vi "observacao_queued.vi"() -> ()   [LabVIEW 2012, in "Shared_160.lvlib"] (continued)
                        n2703 = Greater?(x=w3327, y=w3326) -> (0:w3321:bool)
                        n2704 = case shown="True" w3321 {
                          frame False {
                          }
                          frame True {
                            n2705 = local write "LED ACTION"(TRUE ("LED ACTION")) -> ()
                          }
                        }
                        n2706 = Select(t="REPOUSO" ("y"), s=w3321, f="ESPERA3" ("y")) -> (s? t:f=w3324:string)
                      }
                      frame "REPOUSO" {
                      }
                    }
                    n2707 = local write "ESTADO ABRIR"(w3268) -> ()
                  }
                }
              }
              frame #2 {
                # "MÁQUINA DE ESTADOS PROTEÇÃO"
                n2708 = case shown="3" "M_PROT" {
                  selector: "M_PROT" -> [w3385 _ _ _ _ _]
                  tunnel: [w3385 w3386 w3405 5 5 ("estadoCUP") 0 ("estadoCUP")] -> w3383
                  frame 0, Default {
                    # "Sem movimento"
                    n2709 = call "TickTimeout.vi"() -> ("msTick"=→"Timeout PROT":u32)  [unwired: 2 in, 2 out]
                  }
                  frame 1 {
                    w3389 = u16 3 items=["Alarme", "Atencao", "Erro", "Ocupado", "Protecao", "Embreagem", "Tracking", "Var. Track", "Rápido", "Ligeiro", "Médio", "Lento", "Em movimento", ""] ("NomeStatus")
                    w3388 = u16 3 items=["Alarme", "Atencao", "Erro", "Ocupado", "Protecao", "Embreagem", "Tracking", "Var. Track", "Rápido", "Ligeiro", "Médio", "Lento", "Em movimento", ""] ("NomeStatus")
                    # "Testa Ocupado"
                    n2710 = call "Bit Status DEC.vi"("NomeStatus"=w3388) -> ("StatBit"=w3390:bool)
                    n2711 = call "Bit Status AH.vi"("NomeStatus"=w3389) -> ("StatBit"=w3391:bool)
                    n2712 = Or(x=w3391, y=w3390) -> (x .or. y?=w3387:bool)
                    n2713 = case shown="False" w3387 {
                      tunnel: [2 w3402] -> w3386
                      frame False {
                        w3398 = u16 2 items=["ZERO", "AH", "DEC", "TUBO", "CUP"] ("Controlador")
                        w3393 = u16 1 items=["ZERO", "AH", "DEC", "TUBO", "CUP"] ("Controlador")
                        # "Comando para os controladores\nsaírem da Proteção"
                        n2714 = call "Monta Comando.vi"("Comando"="LIBERAR", "Dispositivo"="EIXO" ("Comando"), "Controlador"=w3393) -> ()  [unwired: 4 in, 3 out]
                        n2715 = call "Monta Comando.vi"("Comando"="LIBERAR", "Dispositivo"="EIXO" ("Comando"), "Controlador"=w3398) -> ()  [unwired: 4 in, 3 out]
                      }
                      frame True {
                        # "Busy"
                        n2716 = local read "Timeout PROT"() -> (w3401:u32)
                        n2717 = call "TickTimeout.vi"("msInicial"=w3401, "msTimeout"=u32 20000) -> ("Timeout"=w3399:bool)  [unwired: 2 out]
                        n2718 = case shown="False" w3399 {
                          tunnel: [1 3] -> w3402
                          frame False {
                          }
                          frame True {
                          }
                        }
                      }
                    }
                  }
                  frame 2 {
                    # "Cálculos rápidos"
                    # "Vem do Setup"
                    # "Aguarda Sair da proteção"
                    n2719 = global read "Global_Telescopio.vi" "Zenital angle GRAUS"() -> (w3408:dbl)
                    n2720 = global read "Global_Telescopio.vi" "Z_LIBERA_GRAUS"() -> (w3407:dbl)
                    n2721 = Less?(x=w3408, y=w3407) -> (x < y?=w3406:bool)
                    n2722 = case shown="True" w3406 {
                      tunnel: [2 ("estadoCUP") 4 ("estadoCUP")] -> w3405
                      frame False {
                      }
                      frame True {
                        # "stop"
                      }
                    }
                  }
                  frame 3 {
                    w3411 = "TENTE NOVAMENTE" ("SYSTEM MESSAGES")
                    # "Trata Timeout"
                    n2723 = call "TickTimeout.vi"() -> ("msTick"=w3412:u32)  [unwired: 2 in, 2 out]
                    n2724 = call "Monta_Mensagem.vi"("Mensagem"=w3411) -> ()  [unwired: 2 in]
                    n2725 = call "Salva_systems_messages.vi"("Mensagem"=w3411) -> ()  [unwired: 5 in]
                    n2726 = local write "Timeout PROT"(w3412) -> ()
                  }
                  frame 4 {
                    w3415 = u16 1 items=["ZERO", "AH", "DEC", "TUBO", "CUP"] ("Controlador")
                    w3420 = u16 2 items=["ZERO", "AH", "DEC", "TUBO", "CUP"] ("Controlador")
                    # "Para os motores"
                    n2727 = call "Monta Comando.vi"("Comando"="PARAR", "Dispositivo"="PROG", "Controlador"=w3415) -> ()  [unwired: 4 in, 3 out]
                    n2728 = call "Monta Comando.vi"("Comando"="PARAR", "Dispositivo"="PROG", "Controlador"=w3420) -> ()  [unwired: 4 in, 3 out]
                  }
                  frame 5 {
                    # "SAÍDA"
                  }
                }
                n2729 = local write "M_PROT"(w3383) -> ()
              }
              frame #3 {
                w3439 = u16 3 items=["Alarme", "Atencao", "Erro", "Ocupado", "TBD", "LCB", "Trapeira", "Paravento", "DomoRap", "DomoCW", "DomoCCW", "TBD", "Em movimento", "TBD"] ("NomeStatus")
                w3447 = u16 3 items=["Alarme", "Atencao", "Erro", "Ocupado", "Protecao", "Embreagem", "Tracking", "Var. Track", "Rápido", "Ligeiro", "Médio", "Lento", "Em movimento", ""] ("NomeStatus")
                w3448 = u16 3 items=["Alarme", "Atencao", "Erro", "Ocupado", "Protecao", "Embreagem", "Tracking", "Var. Track", "Rápido", "Ligeiro", "Médio", "Lento", "Em movimento", ""] ("NomeStatus")
                n2730 = global read "Global_Telescopio.vi" "LimiarRapMed"() -> (w3449:dbl)
                n2731 = global read "Global_Telescopio.vi" "PosAH"() -> (w3451:dbl)
                n2732 = global read "Global_Telescopio.vi" "ErroMaxEixo"() -> (w3446:dbl)
                n2733 = global read "Global_Telescopio.vi" "PosDEC"() -> (w3450:dbl)
                n2734 = call "Bit Status DEC.vi"("NomeStatus"=w3447) -> ("StatBit"=w3445:bool)
                n2735 = call "Bit Status AH.vi"("NomeStatus"=w3448) -> ("StatBit"=w3444:bool)
                n2736 = case shown="4" "M_DEC" {
                  selector: "M_DEC" -> [w3548 _ _ _ _ _ _ _ _]
                  tunnel: [w3548 w3554 w3581 w3606 w3629 w3653 0 w3670 w3675] -> w3428
                  tunnel: "DestDEC" -> [_ w3553 w3578 w3600 w3626 _ _ _ _]
                  tunnel: w3450 -> [_ w3556 _ w3603 _ _ _ _ _]
                  tunnel: w3446 -> [_ _ _ w3604 _ _ _ _ _]
                  tunnel: w3449 -> [_ w3555 _ _ _ _ _ _ _]
                  tunnel: w3445 -> [_ w3552 _ w3599 _ _ _ _ _]
                  frame 0, Default {
                    w3546 = 0 ("CR DEC")
                    # "Sem apontamento"
                    n2737 = call "TickTimeout.vi"() -> ("msTick"=→"TimeoutDEC 2":u32)  [unwired: 2 in, 2 out]
                    "CR DEC UTILS" <- w3546
                    "CONT DEC UTILS" <- w3546
                  }
                  frame 1 {
                    # "Envia\nComando"
                    n2738 = Subtract(x=w3553, y=w3556) -> (x-y=w3551:dbl)
                    n2739 = Absolute Value(x=w3551) -> (abs(x)=w3557:dbl)
                    n2740 = Less?(x=w3557, y=w3555) -> (x < y?=w3550:bool)
                    n2741 = case shown="False" w3550 {
                      tunnel: [w3561 3] -> w3554
                      tunnel: w3553 -> [w3560 _]
                      tunnel: w3551 -> [w3559 _]
                      tunnel: w3552 -> [w3558 _]
                      frame False {
                        # "destino"
                        # "Fora do"
                        n2742 = case shown="False" w3558 {
                          tunnel: [20 w3570] -> w3561
                          tunnel: w3560 -> [w3564 _]
                          tunnel: w3559 -> [_ _]
                          frame False {
                            w3568 = u16 2 items=["ZERO", "AH", "DEC", "TUBO", "CUP"] ("Controlador")
                            # "CLP Pronto"
                            n2743 = local write "DEC on Target"(FALSE ("DEC on Target")) -> ()
                            n2744 = call "rad_hms.vi"("TRUE=HORA\nFALSE=GRAU"=FALSE, "Radiano"=w3564) -> ("Hora/Graus Texto Decimal"=w3565:string)  [unwired: 3 in]
                            n2745 = call "Monta Comando.vi"("Set Point"=w3565, "Comando"="MOVER_RAP", "Dispositivo"="EIXO" ("Comando"), "Controlador"=w3568) -> ()  [unwired: 3 in, 3 out]
                          }
                          frame True {
                            # "CLP Ocupado"
                            n2746 = local read "TimeoutDEC 2"() -> (w3572:u32)
                            n2747 = call "TickTimeout.vi"("msInicial"=w3572, "msTimeout"=u32 4000) -> ("Timeout"=w3571:bool)  [unwired: 2 out]
                            n2748 = case shown="False" w3571 {
                              tunnel: [1 5] -> w3570
                              frame False {
                              }
                              frame True {
                                # "Tratar\nTimeout"
                              }
                            }
                          }
                        }
                      }
                      frame True {
                        # "Dist. pequena p/ mov. rápido"
                        # "Ligar mov. lento"
                        n2749 = call "TickTimeout.vi"() -> ("msTick"=w3576:u32)  [unwired: 2 in, 2 out]
                        n2750 = local write "TimeoutDEC 2"(w3576) -> ()
                      }
                    }
                    n2751 = local write "dec="(FALSE ("dec=")) -> ()
                  }
                  frame 2 {
                    w3584 = u16 12 items=["Alarme", "Atencao", "Erro", "Ocupado", "Protecao", "Embreagem", "Tracking", "Var. Track", "Rápido", "Ligeiro", "Médio", "Lento", "Em movimento", ""] ("NomeStatus")
                    # "Aguarda fim mov. Rap."
                    n2752 = call "Bit Status DEC.vi"("NomeStatus"=w3584) -> ("StatBit"=w3585:bool)
                    n2753 = case shown="True" w3585 {
                      tunnel: [1 w3594] -> w3582
                      tunnel: w3578 -> [_ w3593]
                      frame False {
                        # "Motor parado.\nTestar se chegou\nao destino"
                        n2754 = call "TickTimeout.vi"() -> ("msTick"=w3590:u32)  [unwired: 2 in, 2 out]
                        n2755 = local write "TimeoutDEC 2"(w3590) -> ()
                      }
                      frame True {
                        # "Ainda movendo...\nAGUARDAR"
                        n2756 = call "PROTECAO_DEC_UTILS.vi"("Destino DEC"=w3593) -> ("CONT DEC"=w3592:i32)  [unwired: 10 in]
                        n2757 = local read "Erro PROTEC"() -> (w3595:i32)
                        n2758 = Greater Or Equal?(x=w3592, y=w3595) -> (x >= y?=w3598:bool)
                        n2759 = local write "CONT DEC UTILS"(w3592) -> ()
                        n2760 = Select(t=6, s=w3598, f=2) -> (s? t:f=w3594:i32)
                      }
                    }
                    n2761 = global read "Global_Telescopio.vi" "Habilita supervisao"() -> (w3580:bool)
                    n2762 = case shown="True" w3580 {
                      tunnel: [FALSE w3589] -> w3579
                      frame False {
                      }
                      frame True {
                        n2763 = local read "CR DEC UTILS"() -> (w3587:i32)
                        n2764 = local read "Erro Lim"() -> (w3588:i32)
                        n2765 = Greater Or Equal?(x=w3587, y=w3588) -> (x >= y?=w3589:bool)
                      }
                    }
                    n2766 = Select(t=6, s=w3579, f=w3582) -> (s? t:f=w3581:i32)
                  }
                  frame 3 {
                    # "Mov.Lento"
                    n2767 = Subtract(x=w3600, y=w3603) -> (x-y=w3601:dbl)
                    n2768 = Absolute Value(x=w3601) -> (abs(x)=w3605:dbl)
                    n2769 = Less Or Equal?(x=w3605, y=w3604) -> (x <= y?=w3602:bool)
                    n2770 = case shown="False" w3602 {
                      tunnel: [w3608 0] -> w3606
                      tunnel: w3601 -> [w3607 _]
                      tunnel: w3599 -> [w3609 _]
                      frame False {
                        n2771 = case shown="False" w3609 {
                          tunnel: [40 w3618] -> w3608
                          tunnel: w3607 -> [w3612 _]
                          frame False {
                            w3617 = u16 2 items=["ZERO", "AH", "DEC", "TUBO", "CUP"] ("Controlador")
                            # "Mov. lento"
                            n2772 = call "TickTimeout.vi"() -> ("msTick"=w3610:u32)  [unwired: 2 in, 2 out]
                            n2773 = local write "TimeoutDEC 2"(w3610) -> ()
                            n2774 = call "rad_hms.vi"("TRUE=HORA\nFALSE=GRAU"=FALSE ("TRUE=HORA\nFALSE=GRAU"), "Radiano"=w3612) -> ("Hora/Graus Texto Decimal"=w3614:string)  [unwired: 3 in]
                            n2775 = call "Monta Comando.vi"("Set Point"=w3614, "Comando"="MOVER_REL", "Dispositivo"="EIXO" ("Comando"), "Controlador"=w3617) -> ()  [unwired: 3 in, 3 out]
                          }
                          frame True {
                            # "CLP Ocupado"
                            n2776 = local read "TimeoutDEC 2"() -> (w3620:u32)
                            n2777 = call "TickTimeout.vi"("msInicial"=w3620, "msTimeout"=u32 2000) -> ("Timeout"=w3619:bool)  [unwired: 2 out]
                            n2778 = case shown="False" w3619 {
                              tunnel: [3 5] -> w3618
                              frame False {
                              }
                              frame True {
                              }
                            }
                          }
                        }
                      }
                      frame True {
                        # "DEC no destino"
                        n2779 = local write "DEC on Target"(TRUE ("DEC on Target")) -> ()
                      }
                    }
                  }
                  frame 4 {
                    w3632 = u16 12 items=["Alarme", "Atencao", "Erro", "Ocupado", "Protecao", "Embreagem", "Tracking", "Var. Track", "Rápido", "Ligeiro", "Médio", "Lento", "Em movimento", ""] ("NomeStatus")
                    # "Aguarda fim mov. lento"
                    n2780 = call "Bit Status DEC.vi"("NomeStatus"=w3632) -> ("StatBit"=w3633:bool)
                    n2781 = case shown="True" w3633 {
                      tunnel: [3 w3643] -> w3628
                      tunnel: w3626 -> [_ w3641]
                      frame False {
                        # "Motor parado.\nTestar se chegou\nao destino"
                        n2782 = call "TickTimeout.vi"() -> ("msTick"=w3638:u32)  [unwired: 2 in, 2 out]
                        n2783 = local write "TimeoutDEC 2"(w3638) -> ()
                      }
                      frame True {
                        n2784 = call "PROTECAO_DEC_UTILS.vi"("Destino DEC"=w3641) -> ("CONT DEC"=w3640:i32)  [unwired: 10 in]
                        n2785 = local read "Erro PROTEC"() -> (w3646:i32)
                        n2786 = local write "CONT DEC UTILS"(w3640) -> ()
                        n2787 = Greater Or Equal?(x=w3640, y=w3646) -> (x >= y?=w3648:bool)
                        n2788 = local read "TimeoutDEC 2"() -> (w3642:u32)
                        n2789 = call "TickTimeout.vi"("msInicial"=w3642, "msTimeout"=u32 4000) -> ("Timeout"=w3645:bool)  [unwired: 2 out]
                        n2790 = case shown="False" w3645 {
                          tunnel: [4 5] -> w3649
                          frame False {
                          }
                          frame True {
                          }
                        }
                        n2791 = Select(t=6, s=w3648, f=w3649) -> (s? t:f=w3643:i32)
                      }
                    }
                    n2792 = global read "Global_Telescopio.vi" "Habilita supervisao"() -> (w3631:bool)
                    n2793 = case shown="True" w3631 {
                      tunnel: [FALSE w3637] -> w3627
                      frame False {
                      }
                      frame True {
                        n2794 = local read "CR DEC UTILS"() -> (w3635:i32)
                        n2795 = local read "Erro Lim"() -> (w3636:i32)
                        n2796 = Greater Or Equal?(x=w3635, y=w3636) -> (x >= y?=w3637:bool)
                      }
                    }
                    n2797 = Select(t=6, s=w3627, f=w3628) -> (s? t:f=w3629:i32)
                  }
                  frame 5 {
                    w3659 = u16 2 items=["ZERO", "AH", "DEC", "TUBO", "CUP"] ("Controlador")
                    # "Reiniciar apontamento"
                    # "Trata Timeout"
                    n2798 = call "TickTimeout.vi"() -> ("msTick"=w3652:u32)  [unwired: 2 in, 2 out]
                    n2799 = local write "TimeoutDEC 2"(w3652) -> ()
                    n2800 = call "Monta Comando.vi"("Comando"="PARAR", "Dispositivo"="PROG" ("Comando"), "Controlador"=w3659) -> ("Erro Comunicação"=w3654:bool)  [unwired: 4 in, 2 out]
                    n2801 = Select(t=6, s=w3654, f=1) -> (s? t:f=w3653:i32)
                  }
                  frame 6 {
                    n2802 = stacked-sequence {
                      frame #0 {
                        w3664 = u16 2 items=["ZERO", "AH", "DEC", "TUBO", "CUP"] ("Controlador")
                        # "Trata Timeout"
                        n2803 = local write "dec="(TRUE ("dec=")) -> ()
                        n2804 = call "Monta Comando.vi"("Comando"="PARAR", "Dispositivo"="PROG" ("Comando"), "Controlador"=w3664) -> ()  [unwired: 4 in, 3 out]
                      }
                      frame #1 {
                        w3666 = "Erro de Controlador DEC , REAPONTAR !" ("Mensagem")
                        n2805 = local write "Flag de erro p/ apagar lampada"(TRUE ("Flag de erro p/ apagar lampada")) -> ()
                        n2806 = call "Monta_Mensagem.vi"("Mensagem"=w3666) -> ()  [unwired: 2 in]
                        n2807 = call "Salva_systems_messages.vi"("Mensagem"=w3666) -> ()  [unwired: 5 in]
                      }
                      frame #2 {
                        w3668 = u16 2 items=["ZERO", "AH", "DEC", "TUBO", "CUP"] ("Controlador")
                        # "Em movimento não aceita reset"
                        # "Segundo PARAR por garantia"
                        n2808 = call "Monta Comando.vi"("Comando"="PARAR", "Dispositivo"="PROG", "Controlador"=w3668) -> ()  [unwired: 4 in, 3 out]
                      }
                    }
                  }
                  frame 20 {
                    # "Espera entrar\nem movimento"
                    n2809 = local read "Flag ativo DEC"() -> (w3671:bool)
                    n2810 = case shown="True" w3671 {
                      tunnel: [20 ("t") 2 ("t")] -> w3670
                      frame False {
                      }
                      frame True {
                        # "limpa flag"
                        n2811 = local write "Flag ativo DEC"(FALSE ("Flag ativo AH")) -> ()
                      }
                    }
                  }
                  frame 40 {
                    # "Espera entrar\nem movimento"
                    n2812 = local read "Flag ativo DEC"() -> (w3676:bool)
                    n2813 = case shown="True" w3676 {
                      tunnel: [40 ("t") 4 ("t")] -> w3675
                      frame False {
                      }
                      frame True {
                        # "limpa flag"
                        n2814 = local write "Flag ativo DEC"(FALSE ("Flag ativo AH")) -> ()
                      }
                    }
                  }
                }
                n2815 = case shown="1" "M_AH" {
                  selector: "M_AH" -> [w3682 _ _ _ _ _ _ _ _ _ _]
                  tunnel: [w3682 w3683 w3703 w3734 5 w3757 w3786 w3808 0 w3826 w3831] -> w3430
                  tunnel: "DestAH" -> [_ _ w3700 w3730 _ w3753 w3782 _ _ _ _]
                  tunnel: w3451 -> [_ _ w3706 _ _ w3759 _ _ _ _ _]
                  tunnel: w3446 -> [_ _ _ _ _ w3758 _ _ _ _ _]
                  tunnel: w3449 -> [_ _ w3707 _ _ _ _ _ _ _ _]
                  tunnel: w3444 -> [_ w3684 w3701 _ _ w3755 _ _ _ _ _]
                  frame 0, Default {
                    w3680 = 0 ("CR AH")
                    # "Sem apontamento"
                    n2816 = call "TickTimeout.vi"() -> ("msTick"=→"TimeoutAH 2":u32)  [unwired: 2 in, 2 out]
                    "CR AH UTILS" <- w3680
                    "CONT AH UTILS" <- w3680
                  }
                  frame 1 {
                    n2817 = case shown="False" w3684 {
                      tunnel: [2 w3694] -> w3683
                      frame False {
                        n2818 = stacked-sequence {
                          frame #0 {
                            w3689 = u16 1 items=["ZERO", "AH", "DEC", "TUBO", "CUP"] ("Controlador")
                            # "Desliga Acomp Sideral"
                            n2819 = call "Monta Comando.vi"("Comando"="DESLIGAR", "Dispositivo"="SIDERAL" ("Comando"), "Controlador"=w3689) -> ()  [unwired: 4 in, 3 out]
                          }
                          frame #1 {
                            w3692 = u16 1 items=["ZERO", "AH", "DEC", "TUBO", "CUP"] ("Controlador")
                            # "Parar Eixo AH"
                            n2820 = call "Monta Comando.vi"("Comando"="PARAR", "Dispositivo"="PROG" ("Comando"), "Controlador"=w3692) -> ()  [unwired: 4 in, 3 out]
                          }
                        }
                        n2821 = call "TickTimeout.vi"() -> ("msTick"=w3685:u32)  [unwired: 2 in, 2 out]
                        n2822 = local write "TimeoutAH 2"(w3685) -> ()
                      }
                      frame True {
                        n2823 = local read "TimeoutAH 2"() -> (w3693:u32)
                        n2824 = call "TickTimeout.vi"("msInicial"=w3693, "msTimeout"=u32 5000) -> ("Timeout"=w3696:bool)  [unwired: 2 out]
                        n2825 = case shown="False" w3696 {
                          tunnel: [1 7] -> w3694
                          frame False {
                          }
                          frame True {
                          }
                        }
                      }
                    }
                  }
                  frame 2 {
                    # "Mov.Rapido"
                    n2826 = Subtract(x=w3700, y=w3706) -> (x-y=w3704:dbl)
                    n2827 = Absolute Value(x=w3704) -> (abs(x)=w3705:dbl)
                    n2828 = Less?(x=w3705, y=w3707) -> (x < y?=w3702:bool)
                    n2829 = case shown="False" w3702 {
                      tunnel: w3700 -> [w3708 _]
                      tunnel: w3704 -> [_ _]
                      tunnel: [w3709 4] -> w3703
                      tunnel: w3701 -> [w3710 _]
                      frame False {
                        n2830 = case shown="False" w3710 {
                          tunnel: w3708 -> [w3716 _]
                          tunnel: [w3711 w3722] -> w3709
                          frame False {
                            w3718 = u16 1 items=["ZERO", "AH", "DEC", "TUBO", "CUP"] ("Controlador")
                            # "Aguardar\nfim mov."
                            # "Mov. rápido"
                            n2831 = local write "RA on Target"(FALSE ("RA on Target")) -> ()
                            n2832 = call "rad_hms.vi"("TRUE=HORA\nFALSE=GRAU"=TRUE ("TRUE=HORA\nFALSE=GRAU"), "Radiano"=w3716) -> ("Hora/Graus Texto Decimal"=w3721:string)  [unwired: 3 in]
                            n2833 = call "Monta Comando.vi"("Set Point"=w3721, "Comando"="MOVER_RAP", "Dispositivo"="EIXO" ("Comando"), "Controlador"=w3718) -> ("Erro Comunicação"=w3712:bool)  [unwired: 3 in, 2 out]
                            n2834 = Select(t=8, s=w3712, f=30) -> (s? t:f=w3711:i32)
                          }
                          frame True {
                            # "CLP Ocupado"
                            n2835 = local read "TimeoutAH 2"() -> (w3724:u32)
                            n2836 = call "TickTimeout.vi"("msInicial"=w3724, "msTimeout"=u32 4000) -> ("Timeout"=w3723:bool)  [unwired: 2 out]
                            n2837 = case shown="True" w3723 {
                              tunnel: [2 7] -> w3722
                              frame False {
                              }
                              frame True {
                                # "Tratar\nTimeout"
                              }
                            }
                          }
                        }
                      }
                      frame True {
                        # "Dist. pequena p/ mov. rápido"
                        n2838 = call "TickTimeout.vi"() -> ("msTick"=w3728:u32)  [unwired: 2 in, 2 out]
                        n2839 = local write "TimeoutAH 2"(w3728) -> ()
                      }
                    }
                    n2840 = local write "ah="(FALSE ("ah=")) -> ()
                  }
                  frame 3 {
                    w3737 = u16 12 items=["Alarme", "Atencao", "Erro", "Ocupado", "Protecao", "Embreagem", "Tracking", "Var. Track", "Rápido", "Ligeiro", "Médio", "Lento", "Em movimento", ""] ("NomeStatus")
                    # "Aguarda fim mov. Rap."
                    n2841 = call "Bit Status AH.vi"("NomeStatus"=w3737) -> ("StatBit"=w3736:bool)
                    n2842 = case shown="True" w3736 {
                      tunnel: [2 w3746] -> w3733
                      tunnel: w3730 -> [_ w3745]
                      frame False {
                        # "Motor parado.\nTestar se precisa\nde novo cmd. \nde mov. rápido"
                        n2843 = call "TickTimeout.vi"() -> ("msTick"=w3742:u32)  [unwired: 2 in, 2 out]
                        n2844 = local write "TimeoutAH 2"(w3742) -> ()
                      }
                      frame True {
                        # "Aqui também \ncaberia um \nTimeout?"
                        # "Ainda movendo...\nAGUARDAR"
                        n2845 = call "PROTECAO_AH_UTILS.vi"("DestinoAH"=w3745) -> ("CONT AH"=w3744:i32)  [unwired: 10 in]
                        n2846 = local read "Erro PROTEC"() -> (w3748:i32)
                        n2847 = local write "CONT AH UTILS"(w3744) -> ()
                        n2848 = Greater Or Equal?(x=w3744, y=w3748) -> (x >= y?=w3749:bool)
                        n2849 = Select(t=8, s=w3749, f=3) -> (s? t:f=w3746:i32)
                      }
                    }
                    n2850 = global read "Global_Telescopio.vi" "Habilita supervisao"() -> (w3732:bool)
                    n2851 = case shown="True" w3732 {
                      tunnel: [FALSE w3741] -> w3731
                      frame False {
                      }
                      frame True {
                        n2852 = local read "Erro Lim"() -> (w3740:i32)
                        n2853 = local read "CR AH UTILS"() -> (w3739:i32)
                        n2854 = Greater Or Equal?(x=w3739, y=w3740) -> (x >= y?=w3741:bool)
                      }
                    }
                    n2855 = Select(t=8, s=w3731, f=w3733) -> (s? t:f=w3734:i32)
                  }
                  frame 4 {
                    # "Não faz nada"
                    n2856 = call "TickTimeout.vi"() -> ("msTick"=w3752:u32)  [unwired: 2 in, 2 out]
                    n2857 = local write "TimeoutAH 2"(w3752) -> ()
                  }
                  frame 5 {
                    # "Mov.Lento"
                    n2858 = Subtract(x=w3753, y=w3759) -> (x-y=w3754:dbl)
                    n2859 = Absolute Value(x=w3754) -> (abs(x)=w3760:dbl)
                    n2860 = Less Or Equal?(x=w3760, y=w3758) -> (x <= y?=w3756:bool)
                    n2861 = case shown="True" w3756 {
                      tunnel: w3754 -> [w3762 _]
                      tunnel: [w3761 0] -> w3757
                      tunnel: w3755 -> [w3763 _]
                      frame False {
                        n2862 = case shown="False" w3763 {
                          tunnel: w3762 -> [w3768 _]
                          tunnel: [w3767 w3774] -> w3761
                          frame False {
                            w3770 = u16 1 items=["ZERO", "AH", "DEC", "TUBO", "CUP"] ("Controlador")
                            # "Envia Cmd. Mov. Lento"
                            n2863 = call "rad_hms.vi"("TRUE=HORA\nFALSE=GRAU"=TRUE ("TRUE=HORA\nFALSE=GRAU"), "Radiano"=w3768) -> ("Hora/Graus Texto Decimal"=w3773:string)  [unwired: 3 in]
                            n2864 = call "Monta Comando.vi"("Set Point"=w3773, "Comando"="MOVER_REL", "Dispositivo"="EIXO" ("Comando"), "Controlador"=w3770) -> ("Erro Comunicação"=w3765:bool)  [unwired: 3 in, 2 out]
                            n2865 = Select(t=8, s=w3765, f=60) -> (s? t:f=w3767:i32)
                          }
                          frame True {
                            # "CLP Ocupado"
                            n2866 = local read "TimeoutAH 2"() -> (w3776:u32)
                            n2867 = call "TickTimeout.vi"("msInicial"=w3776, "msTimeout"=u32 4000) -> ("Timeout"=w3775:bool)  [unwired: 2 out]
                            n2868 = case shown="False" w3775 {
                              tunnel: [5 7] -> w3774
                              frame False {
                              }
                              frame True {
                              }
                            }
                          }
                        }
                      }
                      frame True {
                        # "AH on Target"
                        n2869 = local write "RA on Target"(TRUE ("RA on Target")) -> ()
                      }
                    }
                  }
                  frame 6 {
                    w3789 = u16 12 items=["Alarme", "Atencao", "Erro", "Ocupado", "Protecao", "Embreagem", "Tracking", "Var. Track", "Rápido", "Ligeiro", "Médio", "Lento", "Em movimento", ""] ("NomeStatus")
                    # "Aguarda fim mov. Lento"
                    n2870 = call "Bit Status AH.vi"("NomeStatus"=w3789) -> ("StatBit"=w3788:bool)
                    n2871 = case shown="True" w3788 {
                      tunnel: [5 w3803] -> w3785
                      tunnel: w3782 -> [_ w3797]
                      frame False {
                        # "Motor parado.\nTestar se chegou\nao destino"
                        n2872 = call "TickTimeout.vi"() -> ("msTick"=w3794:u32)  [unwired: 2 in, 2 out]
                        n2873 = local write "TimeoutAH 2"(w3794) -> ()
                      }
                      frame True {
                        n2874 = local read "Erro PROTEC"() -> (w3805:i32)
                        n2875 = call "PROTECAO_AH_UTILS.vi"("DestinoAH"=w3797) -> ("CONT AH"=w3796:i32)  [unwired: 10 in]
                        n2876 = local write "CONT AH UTILS"(w3796) -> ()
                        n2877 = local read "TimeoutAH 2"() -> (w3798:u32)
                        n2878 = Greater Or Equal?(x=w3796, y=w3805) -> (x >= y?=w3799:bool)
                        n2879 = call "TickTimeout.vi"("msInicial"=w3798, "msTimeout"=u32 4000) -> ("Timeout"=w3802:bool)  [unwired: 2 out]
                        n2880 = case shown="False" w3802 {
                          tunnel: [6 7] -> w3800
                          frame False {
                          }
                          frame True {
                            # "Tratar\nTimeout"
                          }
                        }
                        n2881 = Select(t=8, s=w3799, f=w3800) -> (s? t:f=w3803:i32)
                      }
                    }
                    n2882 = global read "Global_Telescopio.vi" "Habilita supervisao"() -> (w3784:bool)
                    n2883 = case shown="True" w3784 {
                      tunnel: [FALSE w3793] -> w3783
                      frame False {
                      }
                      frame True {
                        n2884 = local read "CR AH UTILS"() -> (w3791:i32)
                        n2885 = local read "Erro Lim"() -> (w3792:i32)
                        n2886 = Greater Or Equal?(x=w3791, y=w3792) -> (x >= y?=w3793:bool)
                      }
                    }
                    n2887 = Select(t=8, s=w3783, f=w3785) -> (s? t:f=w3786:i32)
                  }
                  frame 7 {
                    w3813 = u16 1 items=["ZERO", "AH", "DEC", "TUBO", "CUP"] ("Controlador")
                    # "Reiniciar apontamento"
                    # "Trata Timeout"
                    n2888 = call "TickTimeout.vi"() -> ("msTick"=w3812:u32)  [unwired: 2 in, 2 out]
                    n2889 = local write "TimeoutAH 2"(w3812) -> ()
                    n2890 = call "Monta Comando.vi"("Comando"="PARAR", "Dispositivo"="PROG" ("Comando"), "Controlador"=w3813) -> ("Erro Comunicação"=w3809:bool)  [unwired: 4 in, 2 out]
                    n2891 = Select(t=8, s=w3809, f=2) -> (s? t:f=w3808:i32)
                  }
                  frame 8 {
                    n2892 = stacked-sequence {
                      frame #0 {
                        w3818 = u16 1 items=["ZERO", "AH", "DEC", "TUBO", "CUP"] ("Controlador")
                        # "Reiniciar apontamento"
                        # "Trata Timeout"
                        n2893 = local write "ah="(TRUE ("ah=")) -> ()
                        n2894 = call "Monta Comando.vi"("Comando"="PARAR", "Dispositivo"="PROG" ("Comando"), "Controlador"=w3818) -> ()  [unwired: 4 in, 3 out]
                      }
                      frame #1 {
                        w3822 = "Erro de Controlador RA , REAPONTAR !" ("Mensagem")
                        n2895 = local write "Flag de erro p/ apagar lampada"(TRUE ("Flag de erro p/ apagar lampada")) -> ()
                        n2896 = call "Monta_Mensagem.vi"("Mensagem"=w3822) -> ()  [unwired: 2 in]
                        n2897 = call "Salva_systems_messages.vi"("Mensagem"=w3822) -> ()  [unwired: 5 in]
                      }
                      frame #2 {
                        w3825 = u16 1 items=["ZERO", "AH", "DEC", "TUBO", "CUP"] ("Controlador")
                        # "Em movimento não aceita reset"
                        # "Segundo PARAR por garantia"
                        n2898 = call "Monta Comando.vi"("Comando"="PARAR", "Dispositivo"="PROG", "Controlador"=w3825) -> ()  [unwired: 4 in, 3 out]
                      }
                    }
                  }
                  frame 30 {
                    # "Espera entrar\nem movimento"
                    n2899 = local read "Flag ativo AH"() -> (w3827:bool)
                    n2900 = case shown="True" w3827 {
                      tunnel: [30 ("t") 3 ("t")] -> w3826
                      frame False {
                      }
                      frame True {
                        # "limpa flag"
                        n2901 = local write "Flag ativo AH"(FALSE ("Flag ativo AH")) -> ()
                      }
                    }
                  }
                  frame 60 {
                    # "Espera entrar\nem movimento"
                    n2902 = local read "Flag ativo AH"() -> (w3832:bool)
                    n2903 = case shown="True" w3832 {
                      tunnel: [60 ("t") 6 ("t")] -> w3831
                      frame False {
                      }
                      frame True {
                        # "limpa flag"
                        n2904 = local write "Flag ativo AH"(FALSE ("Flag ativo AH")) -> ()
                      }
                    }
                  }
                }
                n2905 = call "PROTECAO.vi"("Estado In"=w3428) -> ("Estado Out"=w3427:i32)  [unwired: 2 in]
                n2906 = call "PROTECAO.vi"("Estado In"=w3430) -> ("Estado Out"=w3429:i32)  [unwired: 2 in]
                n2907 = local write "M_DEC"(w3427) -> ()
                n2908 = property on="Setup, Pointing & Guiding" class="TabCtl (strict)"() -> ("Page Selector Visible"=w3434:bool)  [unwired: 2 in, 2 out]
                n2909 = local write "M_AH"(w3429) -> ()
                n2910 = global read "Global_Telescopio.vi" "PosCUP"() -> (w3442:i16)
                n2911 = global read "Global_Telescopio.vi" "ErroMaxCup"() -> (w3441:i16)
                n2912 = local read "M_PROT"() -> (w3424:i32)
                n2913 = call "Bit Status CUP.vi"("NomeStatus"=w3439) -> ("StatBit"=w3443:bool)
                n2914 = Not(x=w3434) -> (.not. x?=w3432:bool)
                n2915 = case shown="5" "M_CUP" {
                  selector: "M_CUP" -> [w3456 _ _ _ _ _ _ _ _]
                  tunnel: [w3456 w3457 w3488 1 w3500 w3517 w3522 w3539 0 ("estadoCUP")] -> w3426
                  tunnel: w3443 -> [_ w3459 _ _ w3499 _ w3523 _ _]
                  tunnel: w3442 -> [_ w3463 _ _ _ _ _ _ _]
                  tunnel: "DestCUP" -> [_ w3458 _ _ _ _ _ _ _]
                  tunnel: w3441 -> [_ w3461 _ _ _ _ _ _ _]
                  frame 0, Default {
                    # "Sem movimento"
                    n2916 = call "TickTimeout.vi"() -> ("msTick"=→"TimeoutCUP 2":u32)  [unwired: 2 in, 2 out]
                  }
                  frame 1 {
                    # "Envia\nComando"
                    n2917 = Subtract(x=w3458, y=w3463) -> (x-y=w3462:i16)
                    n2918 = Absolute Value(x=w3462) -> (abs(x)=w3464:i16)
                    n2919 = Less Or Equal?(x=w3464, y=w3461) -> (x <= y?=w3460:bool)
                    n2920 = case shown="True" w3460 {
                      tunnel: w3459 -> [w3467 _]
                      tunnel: w3458 -> [w3466 _]
                      tunnel: [w3465 w3482] -> w3457
                      frame False {
                        # "CUP fora pos."
                        n2921 = case shown="True" w3467 {
                          tunnel: w3466 -> [w3475 _]
                          tunnel: [2 w3476] -> w3465
                          frame False {
                            w3470 = u16 4 items=["ZERO", "AH", "DEC", "TUBO", "CUP"] ("Controlador")
                            # "CLP Pronto"
                            n2922 = Number To Decimal String(number=w3475) -> (decimal integer string=w3474:string)  [unwired: 1 in]
                            n2923 = call "TickTimeout.vi"() -> ("msTick"=w3469:u32)  [unwired: 2 in, 2 out]
                            n2924 = local write "Dome on Target"(FALSE ("Dome on Target")) -> ()
                            n2925 = local write "TimeoutCUP 2"(w3469) -> ()
                            n2926 = call "Monta Comando.vi"("Set Point"=w3474, "Comando"="MOVER", "Dispositivo"="DOMO" ("Comando"), "Controlador"=w3470) -> ()  [unwired: 3 in, 3 out]
                          }
                          frame True {
                            # "CLP Busy"
                            n2927 = local read "TimeoutCUP 2"() -> (w3478:u32)
                            n2928 = call "TickTimeout.vi"("msInicial"=w3478, "msTimeout"=u32 5000) -> ("Timeout"=w3477:bool)  [unwired: 2 out]
                            n2929 = case shown="True" w3477 {
                              tunnel: [1 3] -> w3476
                              frame False {
                              }
                              frame True {
                              }
                            }
                          }
                        }
                      }
                      frame True {
                        # "Verifica\nTrapeira e\nParavento"
                        # "CUP no destino"
                        n2930 = global read "Global_Telescopio.vi" "Parking"() -> (w3485:bool)
                        n2931 = call "TickTimeout.vi"() -> ("msTick"=w3486:u32)  [unwired: 2 in, 2 out]
                        n2932 = local write "TimeoutCUP 2"(w3486) -> ()
                        n2933 = Select(t=4, s=w3485, f=8) -> (s? t:f=w3482:i32)
                      }
                    }
                  }
                  frame 2 {
                    w3487 = u16 12 items=["Alarme", "Atencao", "Erro", "Ocupado", "TBD", "LCB", "Trapeira", "Paravento", "DomoRap", "DomoCW", "DomoCCW", "TBD", "Em movimento", "TBD"] ("NomeStatus")
                    # "Aqui também caberia um Timeout?"
                    # "Aguarda parada motor"
                    n2934 = call "Bit Status CUP.vi"("NomeStatus"=w3487) -> ("StatBit"=w3489:bool)
                    n2935 = case shown="False" w3489 {
                      tunnel: [1 2] -> w3488
                      frame False {
                        # "Motor parado.\nTestar se chegou\nao destino"
                        n2936 = call "TickTimeout.vi"() -> ("msTick"=w3490:u32)  [unwired: 2 in, 2 out]
                        n2937 = local write "TimeoutCUP 2"(w3490) -> ()
                      }
                      frame True {
                        # "Ainda movendo...\nAGUARDAR"
                      }
                    }
                  }
                  frame 3 {
                    w3496 = u16 4 items=["ZERO", "AH", "DEC", "TUBO", "CUP"] ("Controlador")
                    # "Trata Timeout"
                    n2938 = call "TickTimeout.vi"() -> ("msTick"=w3493:u32)  [unwired: 2 in, 2 out]
                    n2939 = local write "TimeoutCUP 2"(w3493) -> ()
                    n2940 = call "Monta Comando.vi"("Comando"="PARAR", "Dispositivo"="PROG" ("Comando"), "Controlador"=w3496) -> ()  [unwired: 4 in, 3 out]
                  }
                  frame 4 {
                    # "Verifica Trapeira"
                    n2941 = case shown="True" "Case Constant\n(See Context Help) 13" {
                      tunnel: [4 w3502] -> w3500
                      tunnel: w3499 -> [_ w3503]
                      frame False {
                      }
                      frame True {
                        n2942 = case shown="False" w3503 {
                          tunnel: [5 w3508] -> w3502
                          frame False {
                            w3507 = u16 4 items=["ZERO", "AH", "DEC", "TUBO", "CUP"] ("Controlador")
                            # "Fechar Trapeira"
                            # "Aguardar abertura Trap."
                            # "CLP Pronto"
                            n2943 = call "Monta Comando.vi"("Comando"="FECHAR", "Dispositivo"="TRAPEIRA" ("Comando"), "Controlador"=w3507) -> ()  [unwired: 4 in, 3 out]
                          }
                          frame True {
                            # "CLP Busy"
                            n2944 = local read "TimeoutCUP 2"() -> (w3510:u32)
                            n2945 = call "TickTimeout.vi"("msInicial"=w3510, "msTimeout"=u32 5000) -> ("Timeout"=w3509:bool)  [unwired: 2 out]
                            n2946 = case shown="False" w3509 {
                              tunnel: [4 3] -> w3508
                              frame False {
                              }
                              frame True {
                              }
                            }
                          }
                        }
                      }
                    }
                  }
                  frame 5 {
                    w3515 = u16 6 items=["Alarme", "Atencao", "Erro", "Ocupado", "TBD", "LCB", "Trapeira", "Paravento", "DomoRap", "DomoCW", "DomoCCW", "TBD", "Em movimento", "TBD"] ("NomeStatus")
                    # "Aqui também caberia um Timeout?"
                    # "Aguarda Fechamento da Trapeira"
                    # "Também poderia ser testado o bit \"Em movimento\".\nNeste caso o código do \"IF\" deve ser permutado."
                    n2947 = call "Bit Status CUP.vi"("NomeStatus"=w3515) -> ("StatBit"=w3516:bool)
                    n2948 = Not(x=w3516) -> (.not. x?=w3514:bool)
                    n2949 = case shown="True" w3514 {
                      tunnel: [5 6] -> w3517
                      frame False {
                        # "Ainda movendo...\nAGUARDAR"
                      }
                      frame True {
                        # "Trapeira Fechada.\nVerificar Paravento."
                        n2950 = call "TickTimeout.vi"() -> ("msTick"=w3519:u32)  [unwired: 2 in, 2 out]
                        n2951 = local write "TimeoutCUP 2"(w3519) -> ()
                      }
                    }
                  }
                  frame 6 {
                    # "Verifica Paravento"
                    n2952 = case shown="True" "Case Constant\n(See Context Help) 14" {
                      tunnel: w3523 -> [_ w3526]
                      tunnel: [8 w3525] -> w3522
                      frame False {
                        # "Paravento Elevado"
                      }
                      frame True {
                        # "Subir Parav."
                        n2953 = case shown="False" w3526 {
                          tunnel: [7 w3531] -> w3525
                          frame False {
                            w3530 = u16 4 items=["ZERO", "AH", "DEC", "TUBO", "CUP"] ("Controlador")
                            # "Aguardar subida Parav."
                            # "CLP Pronto"
                            n2954 = call "Monta Comando.vi"("Comando"="SUBIR", "Dispositivo"="PARAVENTO" ("Comando"), "Controlador"=w3530) -> ()  [unwired: 4 in, 3 out]
                          }
                          frame True {
                            # "CLP Busy"
                            n2955 = local read "TimeoutCUP 2"() -> (w3533:u32)
                            n2956 = call "TickTimeout.vi"("msInicial"=w3533, "msTimeout"=u32 5000) -> ("Timeout"=w3532:bool)  [unwired: 2 out]
                            n2957 = case shown="False" w3532 {
                              tunnel: [6 3] -> w3531
                              frame False {
                              }
                              frame True {
                              }
                            }
                          }
                        }
                      }
                    }
                  }
                  frame 7 {
                    w3538 = u16 7 items=["Alarme", "Atencao", "Erro", "Ocupado", "TBD", "LCB", "Trapeira", "Paravento", "DomoRap", "DomoCW", "DomoCCW", "TBD", "Em movimento", "TBD"] ("NomeStatus")
                    # "Também poderia ser testado o bit \"Em movimento\".\nNeste caso o código do \"IF\" deve ser permutado."
                    # "Aguarda Subida Paravento"
                    n2958 = call "Bit Status CUP.vi"("NomeStatus"=w3538) -> ("StatBit"=w3540:bool)
                    n2959 = Not(x=w3540) -> (.not. x?=w3537:bool)
                    n2960 = case shown="False" w3537 {
                      tunnel: [7 8] -> w3539
                      frame False {
                        # "Ainda movendo...\nAGUARDAR"
                      }
                      frame True {
                        # "Paravento elevado."
                      }
                    }
                  }
                  frame 8 {
                    # "CUP on target"
                    n2961 = local write "Dome on Target"(TRUE ("Dome on Target")) -> ()
                    n2962 = global write "Global_Telescopio.vi" "Parking"(FALSE) -> ()
                  }
                }
                n2963 = call "PROTECAO.vi"("Estado In"=w3426) -> ("Estado Out"=w3425:i32)  [unwired: 2 in]
                n2964 = Compound Arithmetic op=ADD(w3424, w3425, w3429, w3427) -> (w3435:i32)
                n2965 = Equal To 0?(x=w3435) -> (x = 0?=w3433:bool)
                n2966 = And(x=w3433, y=w3432) -> (x .and. y?=w3431:bool)
                n2967 = case shown="True" w3431 {
                  frame False {
                  }
                  frame True {
                    w3452 = FALSE
                    w3453 = u8 0 ("Disabled")
                    # "DESLIGA TODOS"
                    # "HABILITA TODOS"
                    n2968 = local write "BtUtilZenith"(w3452) -> ()
                    n2969 = local write "BtUtilPark"(w3452) -> ()
                    n2970 = local write "PROTEÇÃO"(w3452) -> ()
                    n2971 = local write "FLAT-FIELD"(w3452) -> ()
                    n2972 = local write "ECASS"(w3452) -> ()
                    n2973 = property on="BtUtilPark" class="Bool (strict)"("Disabled"=w3453) -> ()  [unwired: 2 in, 2 out]
                    n2974 = property on="ECASS" class="Bool (strict)"("Disabled"=w3453) -> ()  [unwired: 2 in, 2 out]
                    n2975 = property on="Setup, Pointing & Guiding" class="TabCtl (strict)"("Page Selector Visible"=TRUE) -> ()  [unwired: 2 in, 2 out]
                    n2976 = property on="BtUtilZenith" class="Bool (strict)"("Disabled"=w3453) -> ()  [unwired: 2 in, 2 out]
                    n2977 = property on="FLAT-FIELD" class="Bool (strict)"("Disabled"=w3453) -> ()  [unwired: 2 in, 2 out]
                    n2978 = property on="PROTEÇÃO" class="Bool (strict)"("Disabled"=w3453) -> ()  [unwired: 2 in, 2 out]
                  }
                }
                n2979 = local write "M_CUP"(w3425) -> ()
              }
              frame #4 {
                n2980 = case shown="True" "GO" {
                  frame False {
                  }
                  frame True {
                    w3840 = u16 3 items=["Alarme", "Atencao", "Erro", "Ocupado", "Protecao", "Embreagem", "Tracking", "Var. Track", "Rápido", "Ligeiro", "Médio", "Lento", "Em movimento", ""] ("NomeStatus")
                    w3841 = u16 3 items=["Alarme", "Atencao", "Erro", "Ocupado", "Protecao", "Embreagem", "Tracking", "Var. Track", "Rápido", "Ligeiro", "Médio", "Lento", "Em movimento", ""] ("NomeStatus")
                    n2981 = call "Bit Status AH.vi"("NomeStatus"=w3841) -> ("StatBit"=w3839:bool)
                    n2982 = call "Bit Status DEC.vi"("NomeStatus"=w3840) -> ("StatBit"=w3838:bool)
                    n2983 = Or(x=w3839, y=w3838) -> (x .or. y?=w3837:bool)
                    n2984 = case shown="False" w3837 {
                      frame False {
                        w3842 = FALSE ("RA on Target")
                        w3860 = u16 1 items=["ZERO", "AH", "DEC", "TUBO", "CUP"] ("Controlador")
                        w3865 = u16 2 items=["ZERO", "AH", "DEC", "TUBO", "CUP"] ("Controlador")
                        w3843 = FALSE ("GO")
                        n2985 = local write "RA on Target"(w3842) -> ()
                        n2986 = local write "DEC on Target"(w3842) -> ()
                        n2987 = global read "Global_Telescopio.vi" "Calagem AH"() -> (w3853:dbl)
                        n2988 = call "Comma_to_Point.vi"("Lat_A"="StrPointObjRA 2") -> ("Saída"=w3847:string)
                        n2989 = call "Comma_to_Point.vi"("Lat_A"="StrPointObjDEC 2") -> ("Saída"=w3844:string)
                        n2990 = global read "Global_Telescopio.vi" "Calagem DEC"() -> (w3852:dbl)
                        n2991 = call "hms_rad.vi"("True = hora"=TRUE, "Texto Graus"=w3847) -> ("radianos"=w3848:dbl)  [unwired: 3 in]
                        n2992 = call "hms_rad.vi"("True = hora"=FALSE, "Texto Graus"=w3844) -> ("radianos"=w3849:dbl)  [unwired: 3 in]
                        n2993 = Add(x=w3848, y=w3853) -> (x+y=w3851:dbl)
                        n2994 = Add(x=w3849, y=w3852) -> (x+y=w3850:dbl)
                        n2995 = local write "GO"(w3843) -> ()
                        n2996 = global write "Global_Telescopio.vi" "ObjCentrado"(w3843) -> ()
                        n2997 = call "rad_hms.vi"("TRUE=HORA\nFALSE=GRAU"=TRUE ("TRUE=HORA\nFALSE=GRAU"), "Radiano"=w3851) -> ("Hora/Graus Texto Decimal"=w3857:string)  [unwired: 3 in]
                        n2998 = call "rad_hms.vi"("TRUE=HORA\nFALSE=GRAU"=FALSE, "Radiano"=w3850) -> ("Hora/Graus Texto Decimal"=w3856:string)  [unwired: 3 in]
                        n2999 = call "Monta Comando.vi"("Set Point"=w3857, "Comando"="MOVER_ABS", "Dispositivo"="EIXO" ("Comando"), "Controlador"=w3860) -> ()  [unwired: 3 in, 3 out]
                        n3000 = call "Monta Comando.vi"("Set Point"=w3856, "Comando"="MOVER_ABS", "Dispositivo"="EIXO" ("Comando"), "Controlador"=w3865) -> ()  [unwired: 3 in, 3 out]
                      }
                      frame True {
                      }
                    }
                  }
                }
              }
            }
          }
        }
      }
      frame #3 {
        # "Desabiita Centragem\ndurante apontamento"
        # "PROCESSO TRACKING"
        # "Comando Via serial do Sist\nAquisição"
        # "CHAVES PAINEL"
        n3001 = local read "FLAT-FIELD"() -> (w3866:bool)
        n3002 = local read "BtUtilZenith"() -> (w3867:bool)
        n3003 = case shown="True" "BtShutterClose" {
          frame False {
          }
          frame True {
            w3911 = u16 3 items=["Alarme", "Atencao", "Erro", "Ocupado", "TBD", "LCB", "Trapeira", "Paravento", "DomoRap", "DomoCW", "DomoCCW", "TBD", "Em movimento", "TBD"] ("NomeStatus")
            n3004 = call "Bit Status CUP.vi"("NomeStatus"=w3911) -> ("StatBit"=w3912:bool)
            n3005 = case shown="False" w3912 {
              selector: w3912 -> [w3913 _]
              frame False {
                w3916 = u16 4 items=["ZERO", "AH", "DEC", "TUBO", "CUP"] ("Controlador")
                n3006 = local write "BtShutterClose"(w3913) -> ()
                n3007 = call "Monta Comando.vi"("Comando"="FECHAR", "Dispositivo"="TRAPEIRA" ("Comando"), "Controlador"=w3916) -> ()  [unwired: 4 in, 3 out]
              }
              frame True {
              }
            }
          }
        }
        n3008 = Or(x=w3867, y=w3866) -> (x .or. y?=w3868:bool)
        n3009 = case shown="True" w3868 {
          frame False {
            w3885 = u16 3 items=["Alarme", "Atencao", "Erro", "Ocupado", "Protecao", "Embreagem", "Tracking", "Var. Track", "Rápido", "Ligeiro", "Médio", "Lento", "Em movimento", ""] ("NomeStatus")
            n3010 = call "Bit Status AH.vi"("NomeStatus"=w3885) -> ("StatBit"=w3884:bool)
            n3011 = case shown="False" "MOUNT" {
              tunnel: w3884 -> [w3887 w3896]
              frame False {
                n3012 = local read "LED MOUNT"() -> (w3888:bool)
                n3013 = Not(x=w3887) -> (.not. x?=w3890:bool)
                n3014 = And(x=w3890, y=w3888) -> (x .and. y?=w3889:bool)
                n3015 = case shown="True" w3889 {
                  frame False {
                  }
                  frame True {
                    w3892 = FALSE
                    w3893 = u16 1 items=["ZERO", "AH", "DEC", "TUBO", "CUP"] ("Controlador")
                    n3016 = call "Monta Comando.vi"("Comando"="DESLIGAR", "Dispositivo"="SIDERAL" ("Comando"), "Controlador"=w3893) -> ()  [unwired: 4 in, 3 out]
                    n3017 = local write "LED MOUNT"(w3892) -> ()
                    n3018 = global write "Global_Telescopio.vi" "ObjCentrado"(w3892) -> ()
                    n3019 = property on="Calagem" class="Bool"("Disabled"=u8 2) -> ()  [unwired: 2 in, 2 out]
                  }
                }
              }
              frame True {
                n3020 = local read "LED MOUNT"() -> (w3897:bool)
                n3021 = Or(x=w3896, y=w3897) -> (x .or. y?=w3898:bool)
                n3022 = case shown="False" w3898 {
                  frame False {
                    w3899 = u16 1 items=["ZERO", "AH", "DEC", "TUBO", "CUP"] ("Controlador")
                    n3023 = call "Monta Comando.vi"("Comando"="LIGAR", "Dispositivo"="SIDERAL" ("Comando"), "Controlador"=w3899) -> ()  [unwired: 4 in, 3 out]
                    "LED MOUNT" <- TRUE
                  }
                  frame True {
                  }
                }
              }
            }
          }
          frame True {
            n3024 = local write "LED MOUNT"(FALSE) -> ()
          }
        }
        n3025 = case shown="True" "Stop All" {
          frame False {
          }
          frame True {
            # "MUDANÇA:\nDesligada chave do\nacompanhamento."
            n3026 = local write "MOUNT"(FALSE ("Led Start/Stop")) -> ()
            n3027 = global write "Global_Telescopio.vi" "STOP ALL"(TRUE ("STOP ALL")) -> ()
          }
        }
        n3028 = case shown="True" "RESTART METEOR" {
          frame False {
          }
          frame True {
            n3029 = call "Teste_Read_Meteorologica.vi"() -> ("Erro"=w3917:bool)  [unwired: 2 in]
            n3030 = local write "Default Met"(w3917) -> ()
          }
        }
        n3031 = global read "Global_Telescopio.vi" "Centragem Via Aquisicao"() -> (w3881:bool)
        n3032 = case shown="True" "STOP" {
          frame False {
          }
          frame True {
            n3033 = stacked-sequence {
              frame #0 {
                n3034 = call "Stop.vi"() -> ()  [unwired: 1 in, 1 out]
              }
              frame #1 {
                w3904 = 0 ("estado")
                n3035 = local write "statDEC"(w3904) -> ()
                n3036 = local write "statAH"(w3904) -> ()
                n3037 = local write "statCUP"(w3904) -> ()
              }
              frame #2 {
                w3905 = 0 ("estado")
                n3038 = local write "M_AH"(w3905) -> ()
                n3039 = local write "M_DEC"(w3905) -> ()
                n3040 = local write "M_CUP"(w3905) -> ()
                n3041 = local write "M_PROT"(w3905) -> ()
              }
              frame #3 {
                n3042 = case shown="True" "Case Constant\n(See Context Help) 15" {
                  frame False {
                  }
                  frame True {
                    w3907 = FALSE
                    n3043 = local write "BtUtilZenith"(w3907) -> ()
                    n3044 = local write "FLAT-FIELD"(w3907) -> ()
                    n3045 = local write "PROTEÇÃO"(w3907) -> ()
                    n3046 = local write "BtUtilPark"(w3907) -> ()
                    n3047 = local write "ECASS"(w3907) -> ()
                  }
                }
              }
              frame #4 {
                n3048 = case shown="True" "LedPointing" {
                  frame False {
                  }
                  frame True {
                    n3049 = local write "LedPointing"(FALSE ("LedPointing")) -> ()
                    n3050 = global write "Global_Telescopio.vi" "Botão GO = STOP"(TRUE ("Botão GO = STOP")) -> ()
                  }
                }
              }
            }
          }
        }
        n3051 = control-ref of="BtTargetPoint"() -> (w3873:refnum<vi>)
        n3052 = And(x="Enable Centragem", y=w3881) -> (x .and. y?=w3880:bool)
        n3053 = property class="Bool"(reference=w3873) -> ("Boolean Text.Text"=w3874:string)  [unwired: 1 in, 2 out]
        n3054 = Or(x="BtOnTatget", y=w3880) -> (x .or. y?=w3876:bool)
        n3055 = Equal?(x=w3874, y="STOP") -> (x = y?=w3872:bool)
        n3056 = Not(x=w3872) -> (.not. x?=w3871:bool)
        n3057 = And(x=w3871, y=w3876) -> (x .and. y?=w3877:bool)
        n3058 = case shown="True" w3877 {
          frame False {
          }
          frame True {
            n3059 = stacked-sequence {
              seq-local: [w3918 _ _ _] -> [_ _ _ w3983]
              seq-local: [_ w3932 _ _] -> [_ _ _ w3984]
              seq-local: [_ _ w3946 _] -> [_ _ _ w3985]
              frame #0 {
                # "Transforma estados lógicos\nnuma string hexadecimal"
                n3060 = local read "Processa Centragem"() -> (w3922:bool)
                n3061 = local read "MOV_IDX_AH"() -> (w3920:bool)
                n3062 = local read "ChkModel"() -> (w3924:bool)
